vi "set_voltage.vi"(8 "error in":errorcluster, 10 "voltage":dbl, 11 "VISA resource name":refnum<visa-resource-name>="COM1") -> (0 "error out":errorcluster, 2 "command":string, 3 "VISA resource name out":refnum<visa-resource-name>)   [LabVIEW 2020]
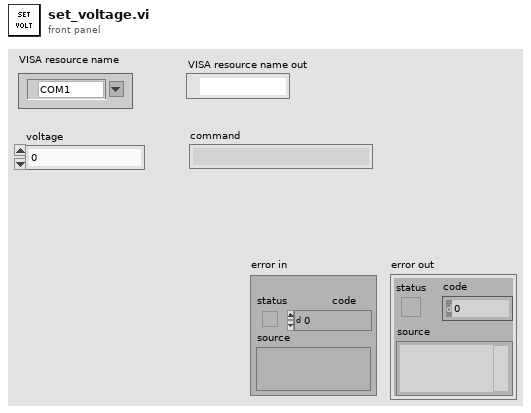
[diagram p1: front panel]
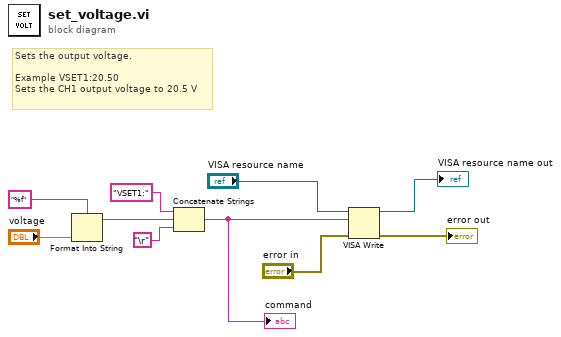
[diagram p0: block diagram]
diagram:
  # "Sets the output voltage.\n\nExample VSET1:20.50\nSets the CH1 output voltage to 20.5 V"
  n1 = Format Into String(format string="%f", "voltage") -> (resulting string=w9:string)  [unwired: 2 in, 1 out]
  n2 = Concatenate Strings("VSET1:" ("string"), w9, "\r") -> (w4:string)
  "command" <- w4
  n3 = VISA Write(VISA resource name="VISA resource name", write buffer=w4, error in (no error)="error in") -> (VISA resource name out=→"VISA resource name out":refnum<visa-resource-name>, error out=→"error out":errorcluster)  [unwired: 1 out]
